vi "FPGA Read Control Scalar Address by Name.vi"(8 "error in (no error)":errorcluster, 9 "Name":string, 10 "Data Type":T1, 11 "FPGA Interface Base in":refnum<class "FPGA Interface Base.lvclass">) -> (0 "error out":errorcluster, 1 "Found?":bool, 2 "Address":u32, 3 "FPGA Interface Base out":refnum<class "FPGA Interface Base.lvclass">)   [LabVIEW 2010, in "FPGA Interface Base.lvclass"]
uses:
  <userlib>/_FPGA Interface Advanced Tools/FPGA Interface Base/FPGA Interface Base.lvclass
  <vilib>/rvi/DataTransferAndStorage/Container/Common/niFpgaDataTypeControl.ctl
  <userlib>/_FPGA Interface Advanced Tools/FPGA Interface Base/FPGA Interface Base.lvclass/FPGA Interface Base.ctl
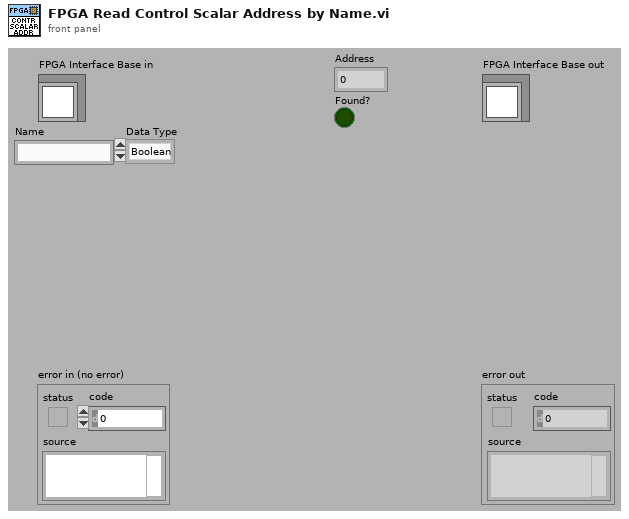
[diagram p1: front panel]
types:
  T1 = typedef "niFpgaDataTypeControl.ctl" = enum32{"Boolean", "I8", "I16", "I32", "I64", "U8", "U16", "U32", "U64", "FXP", "CustomControl"}
  T2 = typedef "FPGA Interface Base.lvclass/FPGA Session.ctl" = refnum<data-value>
  T3 = typedef "FPGA Interface Base.lvclass/FPGA Session Data.ctl" = cluster{"Session Out":u32, "Indicator Scalars":T4, "Indicator Arrays":T6, "Control Scalars":T4, "Control Arrays":T6, "TargetToHost FIFO Channels":T8, "HostToTarget FIFO Channels":T8, "All FIFOs":T9[], "IRQ Context Queue":refnum<queue>}
  T4 = typedef "FPGA Bitfile Utility.lvlib/Scalar Register Set.ctl" = cluster{"Boolean":T5[], "I8":T5[], "I16":T5[], "I32":T5[], "I64":T5[], "U8":T5[], "U16":T5[], "U32":T5[], "U64":T5[]}
  T5 = typedef "FPGA Bitfile Utility.lvlib/Scalar Register.ctl" = cluster{"Address":u32, "Name":string}
  T6 = typedef "FPGA Bitfile Utility.lvlib/Array Register Set.ctl" = cluster{"Boolean":T7[], "I8":T7[], "I16":T7[], "I32":T7[], "I64":T7[], "U8":T7[], "U16":T7[], "U32":T7[], "U64":T7[]}
  T7 = typedef "FPGA Bitfile Utility.lvlib/Array Register.ctl" = cluster{"Address":u32, "Num Elements":u32, "Name":string}
  T8 = typedef "FPGA Bitfile Utility.lvlib/FIFO Channel Set.ctl" = cluster{"Boolean":T9[], "I8":T9[], "I16":T9[], "I32":T9[], "I64":T9[], "U8":T9[], "U16":T9[], "U32":T9[], "U64":T9[]}
  T9 = typedef "FPGA Bitfile Utility.lvlib/FIFO Channel.ctl" = cluster{"Physical Channel":u32, "Name":string}
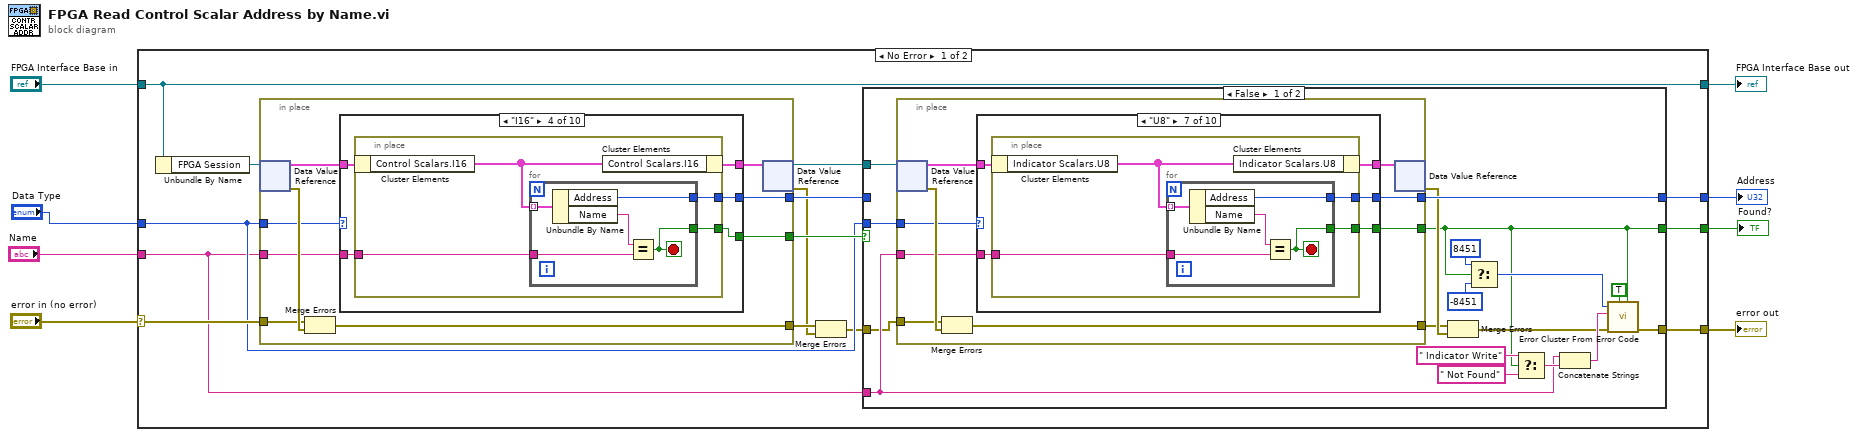
[diagram p0: block diagram]
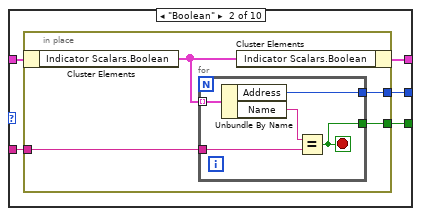
[diagram p3: hidden frame]
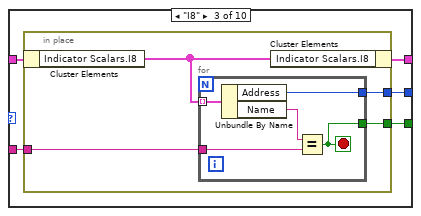
[diagram p4: hidden frame]
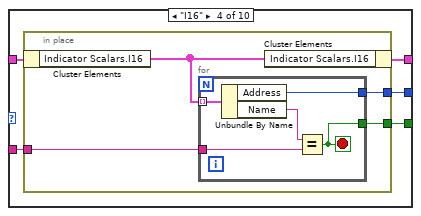
[diagram p5: hidden frame]
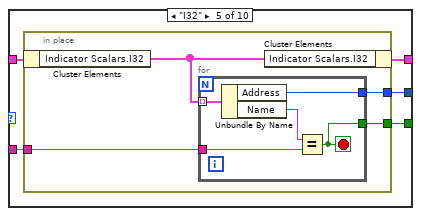
[diagram p6: hidden frame]
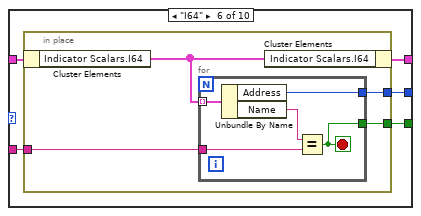
[diagram p7: hidden frame]
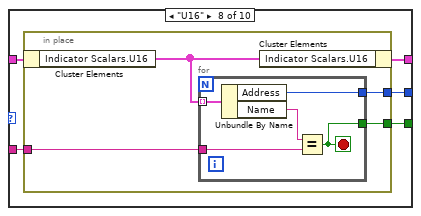
[diagram p8: hidden frame]
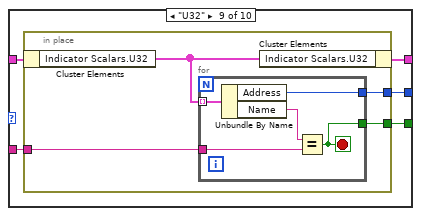
[diagram p9: hidden frame]
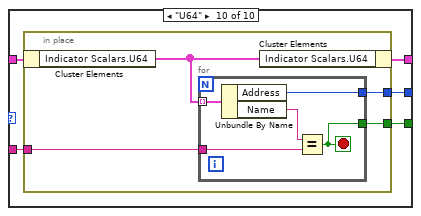
[diagram p10: hidden frame]
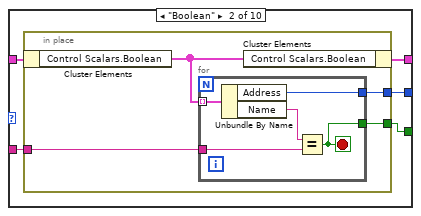
[diagram p13: hidden frame]
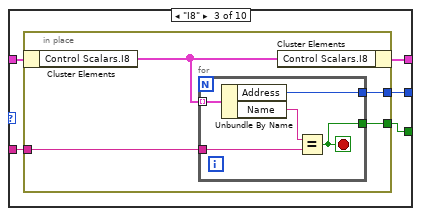
[diagram p14: hidden frame]
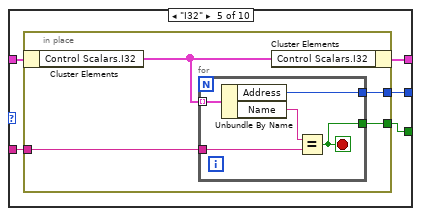
[diagram p15: hidden frame]
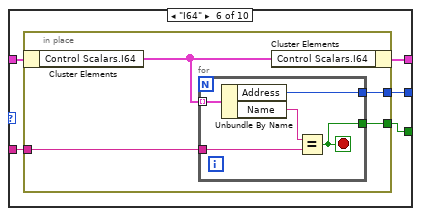
[diagram p16: hidden frame]
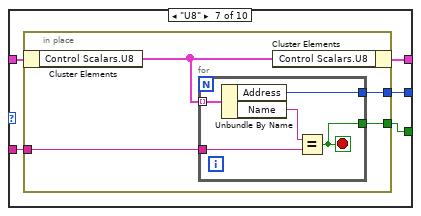
[diagram p17: hidden frame]
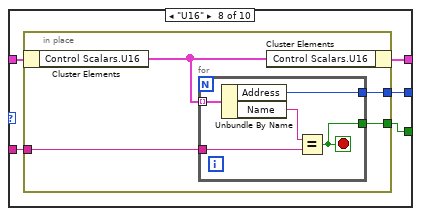
[diagram p18: hidden frame]
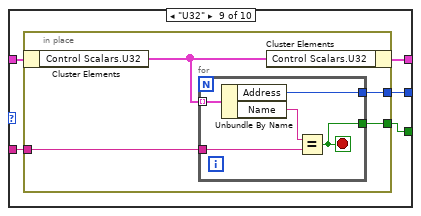
[diagram p19: hidden frame]
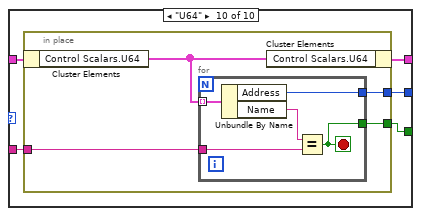
[diagram p20: hidden frame]
diagram:
  n1 = case shown="No Error" "error in (no error)" {
    selector: "error in (no error)" -> [w20 w316]
    tunnel: [w11 w316] -> w7
    tunnel: [w22 w317] -> w5
    tunnel: "FPGA Interface Base in" -> [w22 w317]
    tunnel: [w9 _] -> w4
    tunnel: [w10 _] -> w3
    tunnel: "Name" -> [w15 _]
    tunnel: "Data Type" -> [w16 _]
    frame No Error {
      n2 = Unbundle By Name(w22) -> ("FPGA Session"=w21:T2)
      n3 = in-place {
        in-place-border: w15 -> [w185]
        in-place-border: [w184] -> w18
        in-place-border: [w183] -> w17
        in-place-border: [w182] -> w13
        in-place-border: w20 -> [w181]
        in-place-border: w16 -> [w180]
        n4 = in-place-dvr #1(w21) -> (w187:T3, w188:errorcluster)
        n5 = Merge Errors(w181, w188) -> (w182:errorcluster)
        n6 = case shown="\"I16\"" w180 {
          tunnel: w187 -> [w189 w194 w208 w222 w236 w250 w264 w278 w292 w306]
          tunnel: [w189 w193 w207 w221 w235 w249 w263 w277 w291 w305] -> w186
          tunnel: w185 -> [_ w192 w206 w220 w234 w248 w262 w276 w290 w304]
          tunnel: [_ w191 w205 w219 w233 w247 w261 w275 w289 w303] -> w184
          tunnel: [_ w190 w204 w218 w232 w246 w260 w274 w288 w302] -> w183
          frame Default {
          }
          frame "Boolean" {
            n7 = in-place {
              in-place-border: w192 -> [w197]
              in-place-border: [w196] -> w191
              in-place-border: [w195] -> w190
              n8 = in-place-cluster #2(w194) -> ("Control Scalars.Boolean"=w198:T5[])
              n9 = for {
                tunnel: w198 -> [w203] mode=indexing
                tunnel: [w201] -> w196
                tunnel: [w200] -> w195
                tunnel: w197 -> [w199]
                stop <- w200 stop-if-true
                n10 = Unbundle By Name(w203) -> ("Address"=w201:u32, "Name"=w202:string)
                n11 = Equal?(x=w202, y=w199) -> (x = y?=w200:bool)
              }
              n12 = in-place-cluster #2("Control Scalars.Boolean"=w198) -> (w193:T3)
            }
          }
          frame "I8" {
            n13 = in-place {
              in-place-border: w206 -> [w211]
              in-place-border: [w210] -> w205
              in-place-border: [w209] -> w204
              n14 = in-place-cluster #3(w208) -> ("Control Scalars.I8"=w212:T5[])
              n15 = for {
                tunnel: w212 -> [w217] mode=indexing
                tunnel: [w215] -> w210
                tunnel: [w214] -> w209
                tunnel: w211 -> [w213]
                stop <- w214 stop-if-true
                n16 = Unbundle By Name(w217) -> ("Address"=w215:u32, "Name"=w216:string)
                n17 = Equal?(x=w216, y=w213) -> (x = y?=w214:bool)
              }
              n18 = in-place-cluster #3("Control Scalars.I8"=w212) -> (w207:T3)
            }
          }
          frame "I16" {
            n19 = in-place {
              in-place-border: w220 -> [w225]
              in-place-border: [w224] -> w219
              in-place-border: [w223] -> w218
              n20 = in-place-cluster #4(w222) -> ("Control Scalars.I16"=w226:T5[])
              n21 = for {
                tunnel: w226 -> [w231] mode=indexing
                tunnel: [w229] -> w224
                tunnel: [w228] -> w223
                tunnel: w225 -> [w227]
                stop <- w228 stop-if-true
                n22 = Unbundle By Name(w231) -> ("Address"=w229:u32, "Name"=w230:string)
                n23 = Equal?(x=w230, y=w227) -> (x = y?=w228:bool)
              }
              n24 = in-place-cluster #4("Control Scalars.I16"=w226) -> (w221:T3)
            }
          }
          frame "I32" {
            n25 = in-place {
              in-place-border: w234 -> [w239]
              in-place-border: [w238] -> w233
              in-place-border: [w237] -> w232
              n26 = in-place-cluster #5(w236) -> ("Control Scalars.I32"=w240:T5[])
              n27 = for {
                tunnel: w240 -> [w245] mode=indexing
                tunnel: [w243] -> w238
                tunnel: [w242] -> w237
                tunnel: w239 -> [w241]
                stop <- w242 stop-if-true
                n28 = Unbundle By Name(w245) -> ("Address"=w243:u32, "Name"=w244:string)
                n29 = Equal?(x=w244, y=w241) -> (x = y?=w242:bool)
              }
              n30 = in-place-cluster #5("Control Scalars.I32"=w240) -> (w235:T3)
            }
          }
          frame "I64" {
            n31 = in-place {
              in-place-border: w248 -> [w253]
              in-place-border: [w252] -> w247
              in-place-border: [w251] -> w246
              n32 = in-place-cluster #6(w250) -> ("Control Scalars.I64"=w254:T5[])
              n33 = for {
                tunnel: w254 -> [w259] mode=indexing
                tunnel: [w257] -> w252
                tunnel: [w256] -> w251
                tunnel: w253 -> [w255]
                stop <- w256 stop-if-true
                n34 = Unbundle By Name(w259) -> ("Address"=w257:u32, "Name"=w258:string)
                n35 = Equal?(x=w258, y=w255) -> (x = y?=w256:bool)
              }
              n36 = in-place-cluster #6("Control Scalars.I64"=w254) -> (w249:T3)
            }
          }
          frame "U8" {
            n37 = in-place {
              in-place-border: w262 -> [w267]
              in-place-border: [w266] -> w261
              in-place-border: [w265] -> w260
              n38 = in-place-cluster #7(w264) -> ("Control Scalars.U8"=w268:T5[])
              n39 = for {
                tunnel: w268 -> [w273] mode=indexing
                tunnel: [w271] -> w266
                tunnel: [w270] -> w265
                tunnel: w267 -> [w269]
                stop <- w270 stop-if-true
                n40 = Unbundle By Name(w273) -> ("Address"=w271:u32, "Name"=w272:string)
                n41 = Equal?(x=w272, y=w269) -> (x = y?=w270:bool)
              }
              n42 = in-place-cluster #7("Control Scalars.U8"=w268) -> (w263:T3)
            }
          }
          frame "U16" {
            n43 = in-place {
              in-place-border: w276 -> [w281]
              in-place-border: [w280] -> w275
              in-place-border: [w279] -> w274
              n44 = in-place-cluster #8(w278) -> ("Control Scalars.U16"=w282:T5[])
              n45 = for {
                tunnel: w282 -> [w287] mode=indexing
                tunnel: [w285] -> w280
                tunnel: [w284] -> w279
                tunnel: w281 -> [w283]
                stop <- w284 stop-if-true
                n46 = Unbundle By Name(w287) -> ("Address"=w285:u32, "Name"=w286:string)
                n47 = Equal?(x=w286, y=w283) -> (x = y?=w284:bool)
              }
              n48 = in-place-cluster #8("Control Scalars.U16"=w282) -> (w277:T3)
            }
          }
          frame "U32" {
            n49 = in-place {
              in-place-border: w290 -> [w295]
              in-place-border: [w294] -> w289
              in-place-border: [w293] -> w288
              n50 = in-place-cluster #9(w292) -> ("Control Scalars.U32"=w296:T5[])
              n51 = for {
                tunnel: w296 -> [w301] mode=indexing
                tunnel: [w299] -> w294
                tunnel: [w298] -> w293
                tunnel: w295 -> [w297]
                stop <- w298 stop-if-true
                n52 = Unbundle By Name(w301) -> ("Address"=w299:u32, "Name"=w300:string)
                n53 = Equal?(x=w300, y=w297) -> (x = y?=w298:bool)
              }
              n54 = in-place-cluster #9("Control Scalars.U32"=w296) -> (w291:T3)
            }
          }
          frame "U64" {
            n55 = in-place {
              in-place-border: w304 -> [w309]
              in-place-border: [w308] -> w303
              in-place-border: [w307] -> w302
              n56 = in-place-cluster #10(w306) -> ("Control Scalars.U64"=w310:T5[])
              n57 = for {
                tunnel: w310 -> [w315] mode=indexing
                tunnel: [w313] -> w308
                tunnel: [w312] -> w307
                tunnel: w309 -> [w311]
                stop <- w312 stop-if-true
                n58 = Unbundle By Name(w315) -> ("Address"=w313:u32, "Name"=w314:string)
                n59 = Equal?(x=w314, y=w311) -> (x = y?=w312:bool)
              }
              n60 = in-place-cluster #10("Control Scalars.U64"=w310) -> (w305:T3)
            }
          }
        }
        n61 = in-place-dvr #1(w186) -> (w19:T2, w12:errorcluster)
      }
      n62 = Merge Errors(w13, w12) -> (w14:errorcluster)
      n63 = case shown="False" w17 {
        selector: w17 -> [_ w178]
        tunnel: w19 -> [w30 _]
        tunnel: w14 -> [w23 w177]
        tunnel: w18 -> [_ w179]
        tunnel: [w27 w179] -> w9
        tunnel: [w25 w178] -> w10
        tunnel: [w32 w177] -> w11
        tunnel: w15 -> [w28 _]
        tunnel: w16 -> [w29 _]
        frame False {
          n64 = in-place {
            in-place-border: w28 -> [w46]
            in-place-border: [w45] -> w27
            in-place-border: [w44] -> w25
            in-place-border: [w43] -> w24
            in-place-border: w23 -> [w42]
            in-place-border: w29 -> [w41]
            n65 = in-place-dvr #11(w30) -> (w48:T3, w49:errorcluster)
            n66 = Merge Errors(w42, w49) -> (w43:errorcluster)
            n67 = case shown="\"U8\"" w41 {
              tunnel: w48 -> [w50 w55 w69 w83 w97 w111 w125 w139 w153 w167]
              tunnel: [w50 w54 w68 w82 w96 w110 w124 w138 w152 w166] -> w47
              tunnel: w46 -> [_ w53 w67 w81 w95 w109 w123 w137 w151 w165]
              tunnel: [_ w52 w66 w80 w94 w108 w122 w136 w150 w164] -> w45
              tunnel: [_ w51 w65 w79 w93 w107 w121 w135 w149 w163] -> w44
              frame Default {
              }
              frame "Boolean" {
                n68 = in-place {
                  in-place-border: w53 -> [w58]
                  in-place-border: [w57] -> w52
                  in-place-border: [w56] -> w51
                  n69 = in-place-cluster #12(w55) -> ("Indicator Scalars.Boolean"=w59:T5[])
                  n70 = for {
                    tunnel: w59 -> [w64] mode=indexing
                    tunnel: [w62] -> w57
                    tunnel: [w61] -> w56
                    tunnel: w58 -> [w60]
                    stop <- w61 stop-if-true
                    n71 = Unbundle By Name(w64) -> ("Address"=w62:u32, "Name"=w63:string)
                    n72 = Equal?(x=w63, y=w60) -> (x = y?=w61:bool)
                  }
                  n73 = in-place-cluster #12("Indicator Scalars.Boolean"=w59) -> (w54:T3)
                }
              }
              frame "I8" {
                n74 = in-place {
                  in-place-border: w67 -> [w72]
                  in-place-border: [w71] -> w66
                  in-place-border: [w70] -> w65
                  n75 = in-place-cluster #13(w69) -> ("Indicator Scalars.I8"=w73:T5[])
                  n76 = for {
                    tunnel: w73 -> [w78] mode=indexing
                    tunnel: [w76] -> w71
                    tunnel: [w75] -> w70
                    tunnel: w72 -> [w74]
                    stop <- w75 stop-if-true
                    n77 = Unbundle By Name(w78) -> ("Address"=w76:u32, "Name"=w77:string)
                    n78 = Equal?(x=w77, y=w74) -> (x = y?=w75:bool)
                  }
                  n79 = in-place-cluster #13("Indicator Scalars.I8"=w73) -> (w68:T3)
                }
              }
              frame "I16" {
                n80 = in-place {
                  in-place-border: w81 -> [w86]
                  in-place-border: [w85] -> w80
                  in-place-border: [w84] -> w79
                  n81 = in-place-cluster #14(w83) -> ("Indicator Scalars.I16"=w87:T5[])
                  n82 = for {
                    tunnel: w87 -> [w92] mode=indexing
                    tunnel: [w90] -> w85
                    tunnel: [w89] -> w84
                    tunnel: w86 -> [w88]
                    stop <- w89 stop-if-true
                    n83 = Unbundle By Name(w92) -> ("Address"=w90:u32, "Name"=w91:string)
                    n84 = Equal?(x=w91, y=w88) -> (x = y?=w89:bool)
                  }
                  n85 = in-place-cluster #14("Indicator Scalars.I16"=w87) -> (w82:T3)
                }
              }
              frame "I32" {
                n86 = in-place {
                  in-place-border: w95 -> [w100]
                  in-place-border: [w99] -> w94
                  in-place-border: [w98] -> w93
                  n87 = in-place-cluster #15(w97) -> ("Indicator Scalars.I32"=w101:T5[])
                  n88 = for {
                    tunnel: w101 -> [w106] mode=indexing
                    tunnel: [w104] -> w99
                    tunnel: [w103] -> w98
                    tunnel: w100 -> [w102]
                    stop <- w103 stop-if-true
                    n89 = Unbundle By Name(w106) -> ("Address"=w104:u32, "Name"=w105:string)
                    n90 = Equal?(x=w105, y=w102) -> (x = y?=w103:bool)
                  }
                  n91 = in-place-cluster #15("Indicator Scalars.I32"=w101) -> (w96:T3)
                }
              }
              frame "I64" {
                n92 = in-place {
                  in-place-border: w109 -> [w114]
                  in-place-border: [w113] -> w108
                  in-place-border: [w112] -> w107
                  n93 = in-place-cluster #16(w111) -> ("Indicator Scalars.I64"=w115:T5[])
                  n94 = for {
                    tunnel: w115 -> [w120] mode=indexing
                    tunnel: [w118] -> w113
                    tunnel: [w117] -> w112
                    tunnel: w114 -> [w116]
                    stop <- w117 stop-if-true
                    n95 = Unbundle By Name(w120) -> ("Address"=w118:u32, "Name"=w119:string)
                    n96 = Equal?(x=w119, y=w116) -> (x = y?=w117:bool)
                  }
                  n97 = in-place-cluster #16("Indicator Scalars.I64"=w115) -> (w110:T3)
                }
              }
              frame "U8" {
                n98 = in-place {
                  in-place-border: w123 -> [w128]
                  in-place-border: [w127] -> w122
                  in-place-border: [w126] -> w121
                  n99 = in-place-cluster #17(w125) -> ("Indicator Scalars.U8"=w129:T5[])
                  n100 = for {
                    tunnel: w129 -> [w134] mode=indexing
                    tunnel: [w132] -> w127
                    tunnel: [w131] -> w126
                    tunnel: w128 -> [w130]
                    stop <- w131 stop-if-true
                    n101 = Unbundle By Name(w134) -> ("Address"=w132:u32, "Name"=w133:string)
                    n102 = Equal?(x=w133, y=w130) -> (x = y?=w131:bool)
                  }
                  n103 = in-place-cluster #17("Indicator Scalars.U8"=w129) -> (w124:T3)
                }
              }
              frame "U16" {
                n104 = in-place {
                  in-place-border: w137 -> [w142]
                  in-place-border: [w141] -> w136
                  in-place-border: [w140] -> w135
                  n105 = in-place-cluster #18(w139) -> ("Indicator Scalars.U16"=w143:T5[])
                  n106 = for {
                    tunnel: w143 -> [w148] mode=indexing
                    tunnel: [w146] -> w141
                    tunnel: [w145] -> w140
                    tunnel: w142 -> [w144]
                    stop <- w145 stop-if-true
                    n107 = Unbundle By Name(w148) -> ("Address"=w146:u32, "Name"=w147:string)
                    n108 = Equal?(x=w147, y=w144) -> (x = y?=w145:bool)
                  }
                  n109 = in-place-cluster #18("Indicator Scalars.U16"=w143) -> (w138:T3)
                }
              }
              frame "U32" {
                n110 = in-place {
                  in-place-border: w151 -> [w156]
                  in-place-border: [w155] -> w150
                  in-place-border: [w154] -> w149
                  n111 = in-place-cluster #19(w153) -> ("Indicator Scalars.U32"=w157:T5[])
                  n112 = for {
                    tunnel: w157 -> [w162] mode=indexing
                    tunnel: [w160] -> w155
                    tunnel: [w159] -> w154
                    tunnel: w156 -> [w158]
                    stop <- w159 stop-if-true
                    n113 = Unbundle By Name(w162) -> ("Address"=w160:u32, "Name"=w161:string)
                    n114 = Equal?(x=w161, y=w158) -> (x = y?=w159:bool)
                  }
                  n115 = in-place-cluster #19("Indicator Scalars.U32"=w157) -> (w152:T3)
                }
              }
              frame "U64" {
                n116 = in-place {
                  in-place-border: w165 -> [w170]
                  in-place-border: [w169] -> w164
                  in-place-border: [w168] -> w163
                  n117 = in-place-cluster #20(w167) -> ("Indicator Scalars.U64"=w171:T5[])
                  n118 = for {
                    tunnel: w171 -> [w176] mode=indexing
                    tunnel: [w174] -> w169
                    tunnel: [w173] -> w168
                    tunnel: w170 -> [w172]
                    stop <- w173 stop-if-true
                    n119 = Unbundle By Name(w176) -> ("Address"=w174:u32, "Name"=w175:string)
                    n120 = Equal?(x=w175, y=w172) -> (x = y?=w173:bool)
                  }
                  n121 = in-place-cluster #20("Indicator Scalars.U64"=w171) -> (w166:T3)
                }
              }
            }
            n122 = in-place-dvr #11(w47) -> (w26:errorcluster)  [unwired: 1 out]
          }
          n123 = Merge Errors(w24, w26) -> (w33:errorcluster)
          n124 = Select(t=8451 ("error code (0)"), s=w25, f=-8451 ("error code (0)")) -> (s? t:f=w31:i32)
          n125 = Select(t=" Indicator Write" ("string"), s=w25, f=" Not Found" ("string")) -> (s? t:f=w36:string)
          n126 = Concatenate Strings(w28, w36) -> (w34:string)
          n127 = call <vilib>:"Error Cluster From Error Code.vi"("is warning? (False)"=w25, "show call chain? (False)"=TRUE, "error in (no error)"=w33, "error message (\"\")"=w34, "error code (0)"=w31) -> ("error out"=w32:errorcluster)  [unwired: 4 in]
        }
        frame True {
        }
      }
    }
    frame Error {
    }
  }
  "error out" <- w7
  "FPGA Interface Base out" <- w5
  "Address" <- w4
  "Found?" <- w3
